vi "NanotecSMCPD.get referencing bit.vi"(0 "i ref in":refnum<vi>, 1 "axis":i32, 5 "error in (no error)":errorcluster) -> (14 "i ref out":refnum<vi>, 16 "isReferencing?":bool, 19 "error out":errorcluster)   [LabVIEW 2014, in "NanotecSMCPD.lvlib"]
doc: "Checks, if a reference move is finished. This method does not query the instrument, but decides on the basis of \n\n1) the \"in position\" bit of the status word of the MotorBase class.\n2) the \"referencing\" attribute of THIS class.\n\nFor proper operation, the \"get axis status\" method of THIS class must be executed prior to executing this method."
uses:
  NanotecSMCPD.lvlib
  CSCore/CSSystem/CoreDefs/CoreDefs.error_type.ctl
  CSCore/CSSystem/CoreDefs/CoreDefs.error_severity.ctl
  CSCore/CSApplicationBaseClasses/MotorBase/MotorBase.lvlib
  CSlibraries/UtilityLib/UtilityLib.lvlib
  CSCore/CSSystem/CoreLib/CoreLib.lvlib
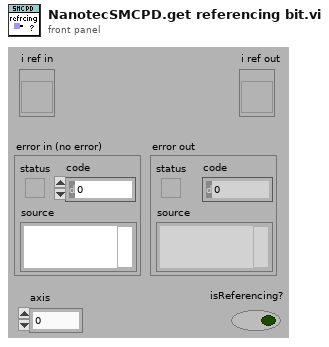
[diagram p1: front panel]
types:
  T1 = typedef "CoreDefs.error_severity.ctl" = enum16{"undefined", "information", "warning", "error", "fatal"}
  T2 = typedef "CoreDefs.error_type.ctl" = enum16{"no error", "can't load process", "can't unload process", "process does not exist", "can't install process", "can't remove process", "unknown function", "time out", "can't execute function", "duplicate queue name", "super not found", "caller queue invalid", "can't ping process", "unknown error", "VISA Error", "VISA timeout", "GPIB timeout", "GPIB error", "communication error", "data type mismatch", "can't read data from OPC server", "can't write data to OPC server", "OET error", "function not implemented", "process already exists", "invalid Shared Variable name", "error writing Shared Variable", "error reading Shared Variable", "invalid client name", "corrupt database", "unknown class", "call not authorized", "parameter out of range", "OET timeout: can't get data to modify", "invalid queue name", "requested operation incompatible with current state", "event undefined", "event disabled", "state undefined", "caller is not a friend", "EventBuilder: bad eventID", "EventBuilder: no DAQ devices", "a thread must not stop itself", "UNUSED ELEMENT4", "DiscArchiver: eventData incomplete", "DiscArchiver: eventData does not belong to run", "DiscArchiver: can't open file", "DiscArchiver: can't write to file", "DiscArchiver: available disc space low", "can't acquire semaphore", "error reading data from database", "notifier object is not existing", "can't register process", "can't unregister process", "illegal event type", "object disabled", "object already exists", "can't change state", "Instrument not found", "no connection to remote node", "invalid reference", "N/A", "UNUSED ELEMENT 1", "element not found", "illegal TCP/IP connection detected", "object does not exist", "invalid access ID", "unknown CS system", "invalid privilige", "unsupported data type", "unsupported server type", "IO server already exists", "Shared Variable already exists"}
  T3 = typedef "NanotecSMCPD.lvlib/NanotecSMCPD.i attribute.ctl" = cluster{"referencing":bool[], "stop":bool[], "AutoHalt ID":i32, "MethodQueue":refnum<queue>, "Referenced1Time?":bool[], "LastCommand ID":i32}
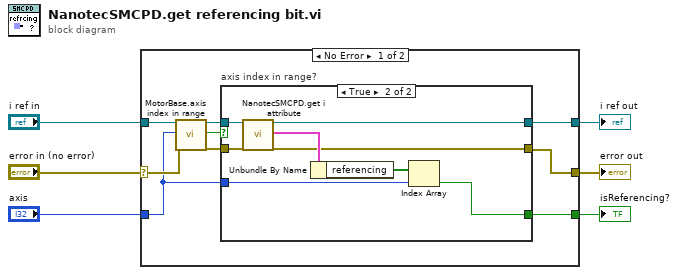
[diagram p0: block diagram]
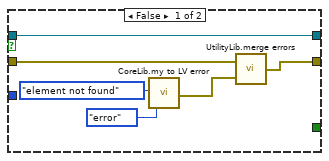
[diagram p2: hidden frame]
diagram:
  n1 = case shown="No Error" "error in (no error)" {
    selector: "error in (no error)" -> [w14 w30]
    tunnel: "i ref in" -> [w15 w31]
    tunnel: [w8 w30] -> w4
    tunnel: [w9 w31] -> w3
    tunnel: "axis" -> [w10 _]
    tunnel: [w7 _] -> w1
    frame No Error {
      n2 = call "MotorBase.axis index in range.vi"("i ref in"=w15, "axisIndex"=w10, "error in (no error)"=w14) -> ("i ref out"=w12:refnum<vi>, "in range"=w11:bool, "error out"=w13:errorcluster)  [unwired: 14 in]
      n3 = case "axis index in range?" shown="True" w11 {
        tunnel: w12 -> [w21 w27]
        tunnel: w13 -> [w20 w28]
        tunnel: [w19 w22] -> w8
        tunnel: w10 -> [_ w26]
        tunnel: [w21 w23] -> w9
        tunnel: [_ w24] -> w7
        frame False {
          n4 = call "CoreLib.my to LV error.vi"("ErrorTypes"=CoreDefs.error_type."element not found", "severityLevel"=CoreDefs.error_severity."error") -> ("myErrorCluster"=w18:errorcluster)  [unwired: 16 in, 1 out]
          n5 = call "UtilityLib.merge errors.vi"("error2 (no error)"=w18, "error1 (no error)"=w20) -> ("error out"=w19:errorcluster)
        }
        frame True {
          n6 = call "NanotecSMCPD.get i attribute.vi"("i ref in"=w27, "error in (no error)"=w28) -> ("i ref out"=w23:refnum<vi>, "i attribute"=w29:T3, "error out"=w22:errorcluster)  [unwired: 15 in]
          n7 = Unbundle By Name(w29) -> ("referencing"=w25:bool[])
          n8 = Index Array(array=w25, index=w26) -> (element=w24:bool)
        }
      }
    }
    frame Error {
    }
  }
  "error out" <- w4
  "i ref out" <- w3
  "isReferencing?" <- w1
